vi "Write To Csv Test.vi"(11 "Error In":errorcluster) -> (15 "Error Out":errorcluster)   [LabVIEW 2021, in "Test Files.lvlib"]
doc: "This VI has test cases for checking the functionality of Write To Csv.vi"
uses:
  Test Files.lvlib
  <vilib>/addons/_JKI Toolkits/Caraya/classes/Test/Test.lvclass
  <vilib>/addons/_JKI Toolkits/Caraya/classes/Assert/Assert.lvclass
  CustomSortPath.lvlib
  <vilib>/addons/_JKI Toolkits/Caraya/classes/Assert/Assert Equal Value_Variant.vi
panel:
  # "Write to CSV file test"
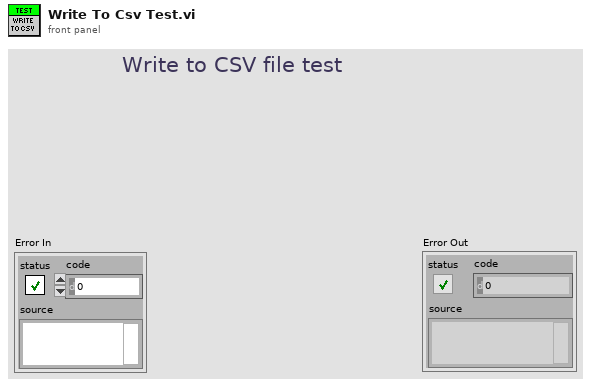
[diagram p1: front panel]
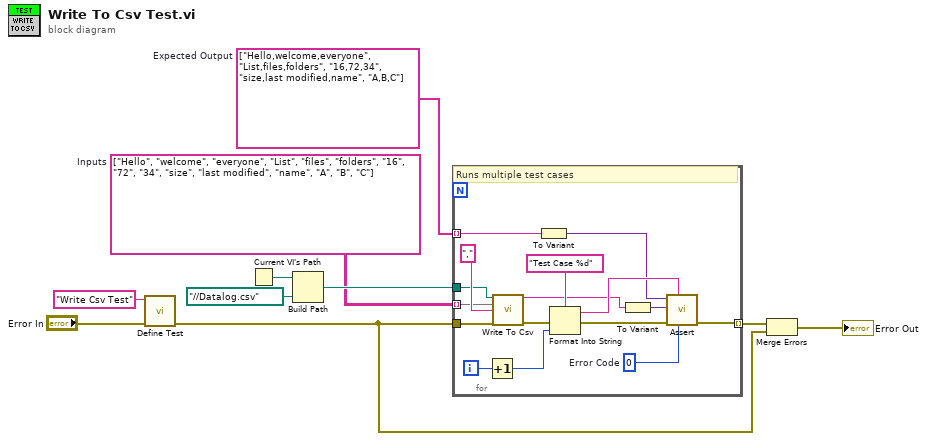
[diagram p0: block diagram]
diagram:
  w5 = string[][] [["Hello", "welcome", "everyone"], ["List", "files", "folders"], ["16", "72", "34"], ["size", "last modified", "name"], ["A", "B", "C"]]  # Inputs
  w4 = string[] ["Hello,welcome,everyone", "List,files,folders", "16,72,34", "size,last modified,name", "A,B,C"]  # Expected Output
  n1 = call <vilib>:"Define Test.vi"("error in (no error)"="Error In", "Label (VI Title)"="Write Csv Test") -> ("error out"=w1:errorcluster)  [unwired: 8 in, 1 out]
  n2 = Current VI's Path() -> (path=w8:path)
  n3 = Build Path(base path=w8, name or relative path=path "../../Datalog.csv") -> (appended path=w6:path)
  n4 = for {
    tunnel: w6 -> [w24]
    tunnel: w5 -> [w23] mode=indexing
    tunnel: w4 -> [w21] mode=indexing
    tunnel: w1 -> [w25]
    tunnel: [w13] -> w3 mode=indexing
    i -> [w18]
    w11 = 0  # Error Code
    # "Runs multiple test cases"
    n5 = Increment(x=w18) -> (x+1=w17:i32)
    n6 = call "Write To Csv.vi"("File Path"=w24, "StringArray"=w23, "delimiter (Tab)"=",", "error in (no error)"=w25) -> ("String Out"=w12:string, "error out"=w22:errorcluster)  [unwired: 10 in]
    n7 = To Variant(anything=w21) -> (Variant=w15:variant)
    n8 = Format Into String(format string="Test Case %d", error in=w22, w17) -> (resulting string=w16:string, error out=w20:errorcluster)  [unwired: 1 in]
    n9 = To Variant(anything=w12) -> (Variant=w14:variant)
    n10 = call-poly <vilib>:"Assert.vi"("error code (1)"=w11, "Label"=w16, "error in (no error)"=w20, "Y"=w14, "X"=w15) -> ("error out"=w13:errorcluster)  [unwired: 5 in, 1 out]
  }
  n11 = Merge Errors(w3, w1) -> (→"Error Out":errorcluster)
